vi "Set Return Values.vi"(8 "error in (no error)":errorcluster, 10 "VI Reference":refnum<vi>, 11 "Mock In":refnum<class "Responsive Mock.lvclass">) -> (0 "error out":errorcluster, 3 "Mock Out":refnum<class "Responsive Mock.lvclass">)   [LabVIEW 2020, in "Responsive Mock.lvclass"]
uses:
  Responsive Mock.lvclass
  Responsive Mock.lvclass/Responsive Mock.ctl
  VI Call/VI Call.lvclass
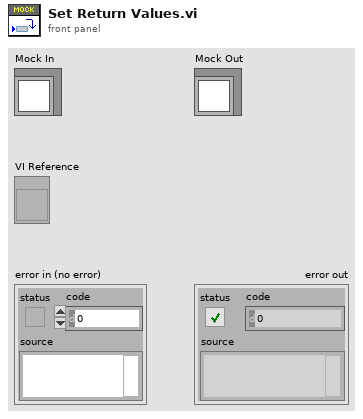
[diagram p1: front panel]
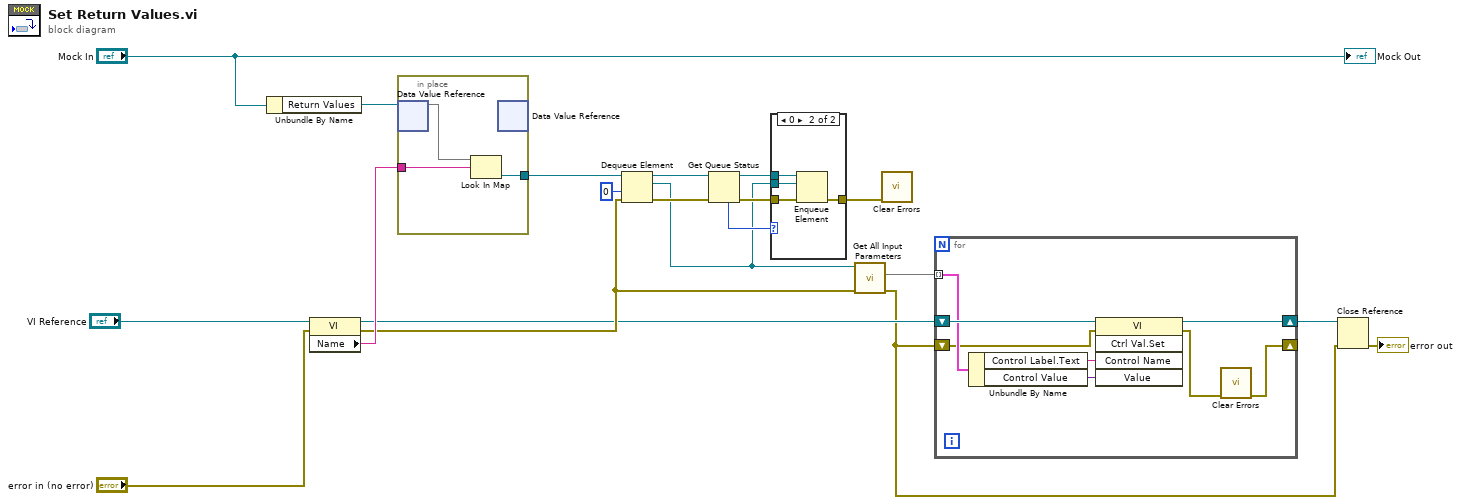
[diagram p0: block diagram]
diagram:
  n1 = Unbundle By Name("Mock In") -> ("Return Values"=w15:refnum<data-value>)
  n2 = property class="VI"(reference="VI Reference", error in="error in (no error)") -> (reference out=w3:refnum<vi>, error out=w5:errorcluster, "Name"=w14:string)
  n3 = in-place {
    in-place-border: w14 -> [w22]
    in-place-border: [w21] -> w13
    n4 = in-place-dvr #1(w15) -> (w23:map{string, refnum<queue>})  [unwired: 1 out]
    n5 = Look In Map(map=w23, key=w22) -> (value=w21:refnum<queue>)  [unwired: 1 in, 1 out]
    n6 = in-place-dvr #1() -> ()  [unwired: 1 in, 2 out]
  }
  n7 = Dequeue Element(queue=w13, timeout in ms (-1)=0, error in (no error)=w5) -> (queue out=w9:refnum<queue>, element=w1:refnum<class "VI Call.lvclass">, error out=w11:errorcluster)  [unwired: 1 out]
  n8 = Get Queue Status(queue=w9, error in (no error)=w11) -> (queue out=w7:refnum<queue>, error out=w10:errorcluster, # elements in queue=w6:i32)  [unwired: 1 in, 5 out]
  n9 = case shown="0" w6 {
    tunnel: w10 -> [w24 w28]
    tunnel: [w24 w27] -> w8
    tunnel: w7 -> [_ w26]
    tunnel: w1 -> [_ w25]
    frame Default {
    }
    frame 0 {
      n10 = Enqueue Element(queue=w26, element=w25, error in (no error)=w28) -> (error out=w27:errorcluster)  [unwired: 1 in, 2 out]
    }
  }
  n11 = call-dynamic "Get All Input Parameters.vi"("error in (no error)"=w5, "VI Call in"=w1) -> ("error out"=w2:errorcluster, "Input Parameters"=w18:map{string, variant})  [unwired: 8 in]
  n12 = call <vilib>:"Clear Errors.vi"("error in (no error)"=w8) -> ()  [unwired: 5 in, 2 out]
  n13 = for {
    tunnel: w18 -> [w35] mode=indexing
    shift-right: [w32] -> w16
    shift-left: w3 -> [w36]
    shift-right: [w29] -> _
    shift-left: w2 -> [w31]
    n14 = Unbundle By Name(w35) -> ("Control Label.Text"=w33:string, "Control Value"=w34:variant)
    n15 = invoke class="VI" method="Ctrl Val.Set"(reference=w36, error in=w31, "Control Name"=w33, "Value"=w34) -> (reference out=w32:refnum<vi>, error out=w30:errorcluster)  [unwired: 1 in, 3 out]
    n16 = call <vilib>:"Clear Errors.vi"("error in (no error)"=w30) -> ("error out"=w29:errorcluster)  [unwired: 5 in, 1 out]
  }
  n17 = Close Reference(reference=w16, error in (no error)=w2) -> (error out=→"error out":errorcluster)
  "Mock Out" <- "Mock In"
